vi "StanleyMethod.vi"(2 "v(Velocity)m/s":dbl, 3 "e(Cross-Track Err)m/s":dbl, 4 "k(Gain)":dbl, 5 "¥÷(Heading Err)radian":dbl) -> (0 "ヤ(OutputSteer)radian":dbl, 1 "ヤ(OutputSteer)degrees":dbl)   [LabVIEW 2024]
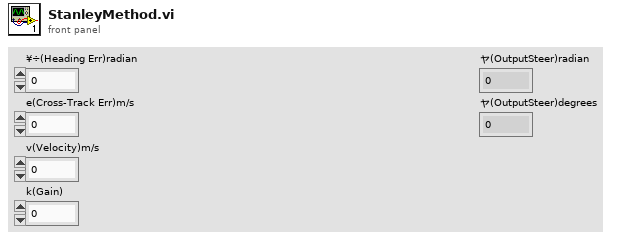
[diagram p1: front panel]
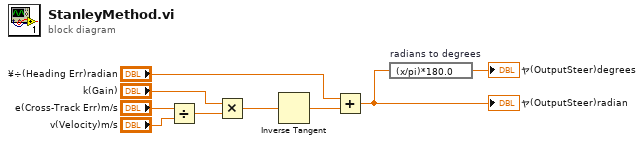
[diagram p0: block diagram]
diagram:
  n1 = Divide(x="e(Cross-Track Err)m/s", y="v(Velocity)m/s") -> (x/y=w6:dbl)
  n2 = Multiply(x="k(Gain)", y=w6) -> (x*y=w7:dbl)
  n3 = Inverse Tangent(1:w7) -> (0:w8:dbl)
  n4 = Add(x="¥÷(Heading Err)radian", y=w8) -> (x+y=w2:dbl)
  "ヤ(OutputSteer)radian" <- w2
  n5 = expression code="(x/pi)*180.0" "radians to degrees"(w2) -> (→"ヤ(OutputSteer)degrees":dbl)
